vi "天气查询.vi"() -> ()   [LabVIEW 2016]
uses:
  Svc_WebService.dll
  <vilib>/regexp/Match Regular Expression.xnode
  <vilib>/httpClient/LabVIEWHTTPClient.lvlib
panel:
  out "子字符串;substring":string
  out "查询结果":string
  in  "城市（市，县）":string
  in  "查询按钮":bool
  out "查询到的整体天气":string[](array[string])
  out "错误输出 2":errorcluster caption="错误输出"
  in  "要查询天气的城市":string
  in  "输入省份查询支持获取天气的城市":string
  out "错误输出":errorcluster
  out "支持查询的城市":string[](array[string])
  in  "错误输入（无错误）":errorcluster
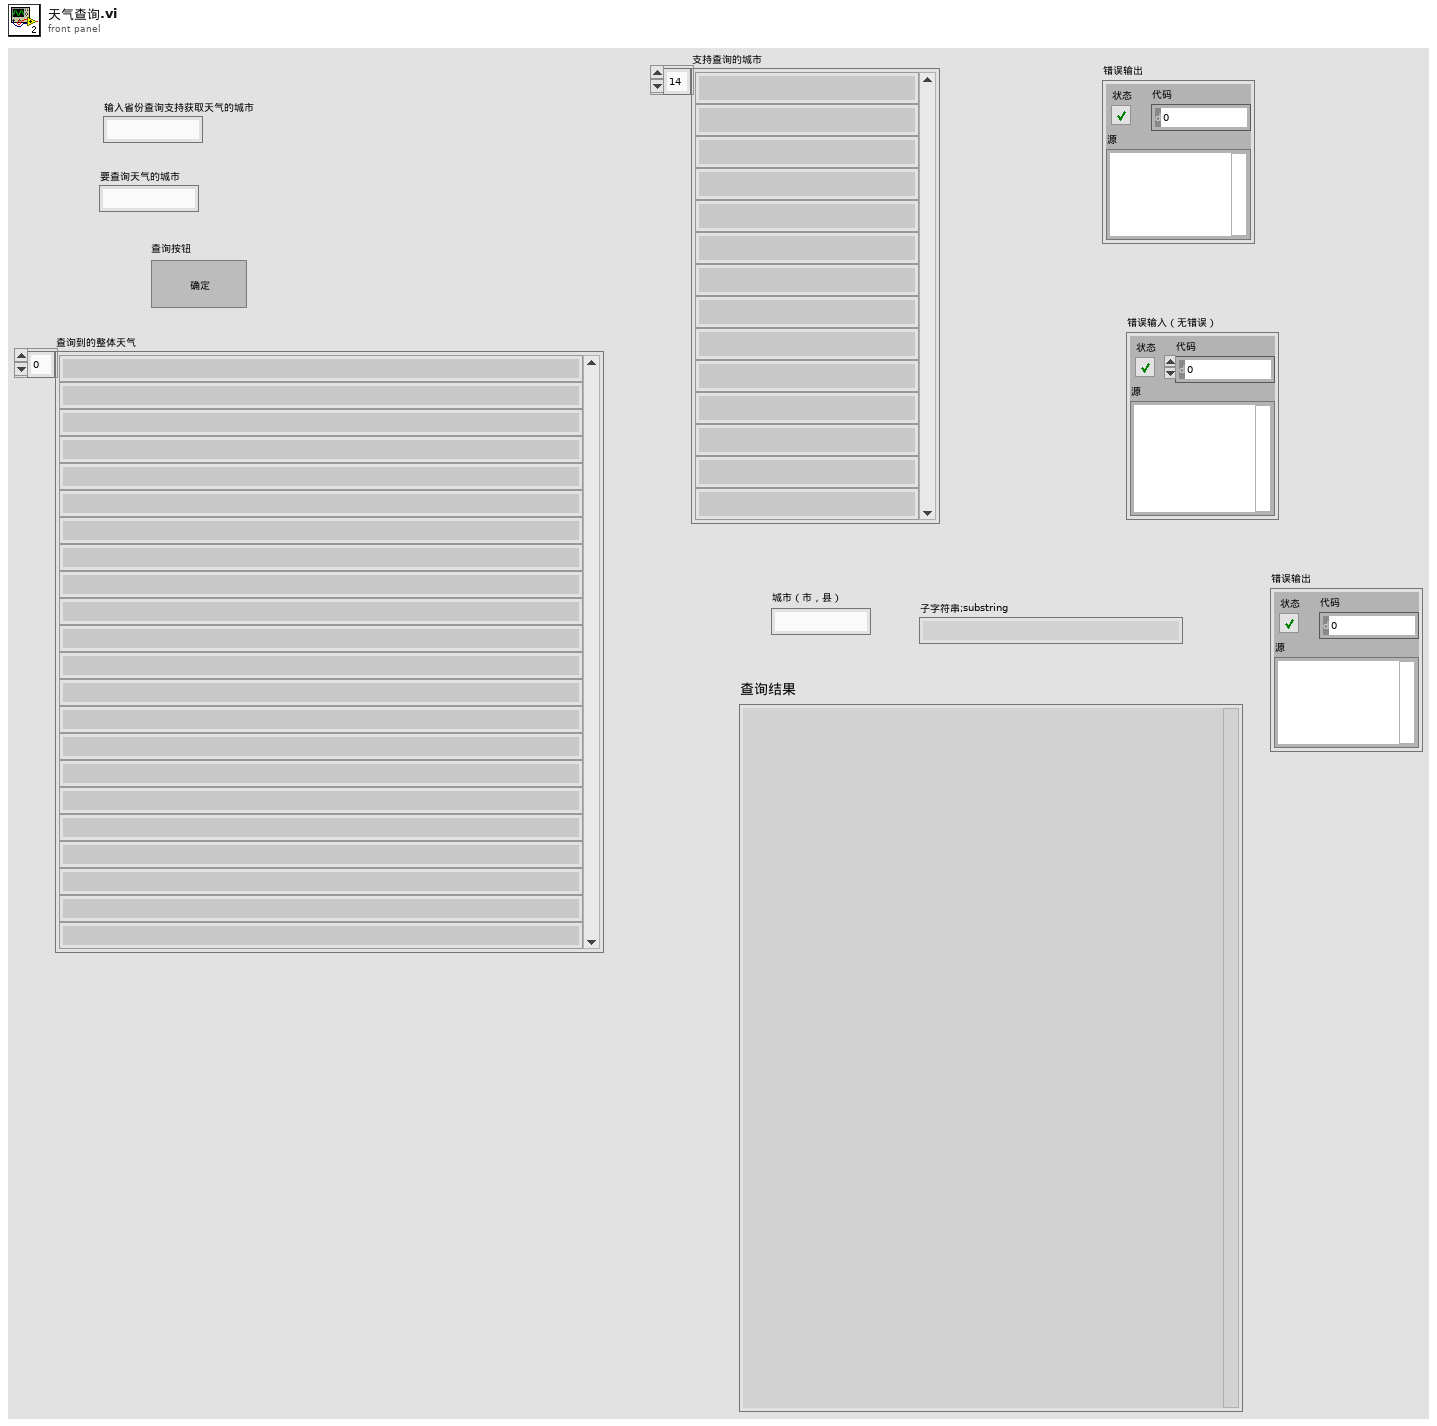
[diagram p1: front panel]
types:
  T1 = typedef "LabVIEWHTTPClient.lvlib/ClientHandle.ctl" = refnum<k1>
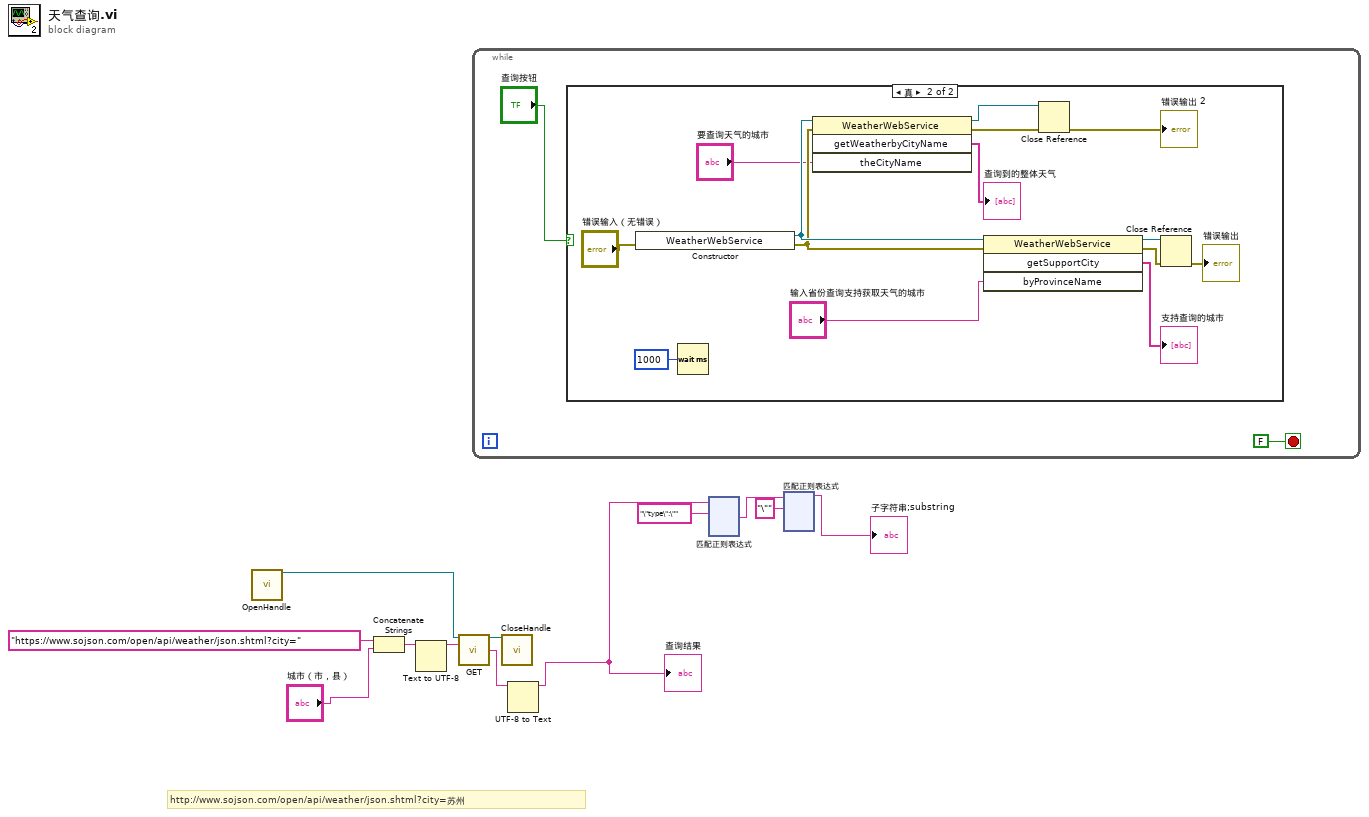
[diagram p0: block diagram]
diagram:
  # "http://www.sojson.com/open/api/weather/json.shtml?city=苏州"
  n1 = call <vilib>:"OpenHandle.vi"() -> ("client handle out"=w7:T1)  [unwired: 14 in, 1 out]
  n2 = Concatenate Strings("https://www.sojson.com/open/api/weather/json.shtml?city=" ("字符串"), "城市（市，县）") -> (w12:string)
  n3 = Text to UTF-8(11:w12) -> (3:w10:string)  [unwired: 2 in, 1 out]
  n4 = call <vilib>:"GET.vi"("client handle"=w7, "url"=w10) -> ("client handle out"=w8:T1, "body"=w9:string)  [unwired: 10 in, 2 out]
  n5 = while {
    stop <- FALSE stop-if-true
    n6 = case shown="真" "查询按钮" {
      frame False {
      }
      frame True {
        n7 = constructor class="WeatherWebService"(error in="错误输入（无错误）") -> (reference out=w22:refnum<k24>, error out=w21:errorcluster)  [unwired: 2 in, 1 out]
        n8 = Wait (ms)(milliseconds to wait=u32 1000 ("等待时间（毫秒）")) -> ()  [unwired: 1 out]
        n9 = invoke on="调用节点" class="WeatherWebService" method="getWeatherbyCityName"(reference=w22, error in=w21, "theCityName"="要查询天气的城市") -> (reference out=w18:refnum<k24>, error out=w17:errorcluster, "getWeatherbyCityName"=→"查询到的整体天气":string[])  [unwired: 1 in, 1 out]
        n10 = invoke on="调用节点" class="WeatherWebService" method="getSupportCity"(reference=w22, error in=w21, "byProvinceName"="输入省份查询支持获取天气的城市") -> (reference out=w25:refnum<k24>, error out=w26:errorcluster, "getSupportCity"=→"支持查询的城市":string[])  [unwired: 1 in, 1 out]
        n11 = Close Reference(reference=w18, error in (no error)=w17) -> (error out=→"错误输出 2":errorcluster)
        n12 = Close Reference(reference=w25, error in (no error)=w26) -> (error out=→"错误输出":errorcluster)
      }
    }
  }
  n13 = call <vilib>:"CloseHandle.vi"("client handle"=w8) -> ()  [unwired: 14 in, 1 out]
  n14 = UTF-8 to Text(11:w9) -> (3:w5:string)  [unwired: 2 in, 1 out]
  "查询结果" <- w5
  n15 = xnode "匹配正则表达式"("输入字符串"=w5, "正则表达式"="\"type\":\"") -> ("匹配之后"=w3:string)  [unwired: 4 in, 4 out]
  n16 = xnode "匹配正则表达式"("输入字符串"=w3, "正则表达式"="\"") -> ("匹配之前"=→"子字符串;substring":string)  [unwired: 4 in, 4 out]
